vi "CRYGet CurrentSteps By StepNo.vi"(11 "Step Setup VI No":i32) -> (0 "bResult":bool, 2 "Index":i32, 3 "Step":T1={"No.VI"=0, "Category"="", "StepName"="", "Seq setup flattened"="", "Comment"="", "Steps config."=[], "Jump config"=[], "Start"=0.0, "Increment"=0.0, "Name"="Pa", "Unit"="Pa", "Y data"=1, "Y prefix"="", "Y dB ref"=1.0, "Y unit"="", "Repeat State Array"=[]} {"Repeat State Array"."Start" format="%#_5g"; "Y dB ref" format="%.1f"; "Y data" items=["dB", "Lin"]; "Start" format="%#_5g"})   [LabVIEW 2013]
uses:
  CRYSystem/Typedef Control/CRYStep.ctl
  CRYProject Editor Global.vi
  CRYCurveLibrary/Global/CRYCurve Library Global.vi
  CRYSystem/Calibration/SubVI/CRYCal Global.vi
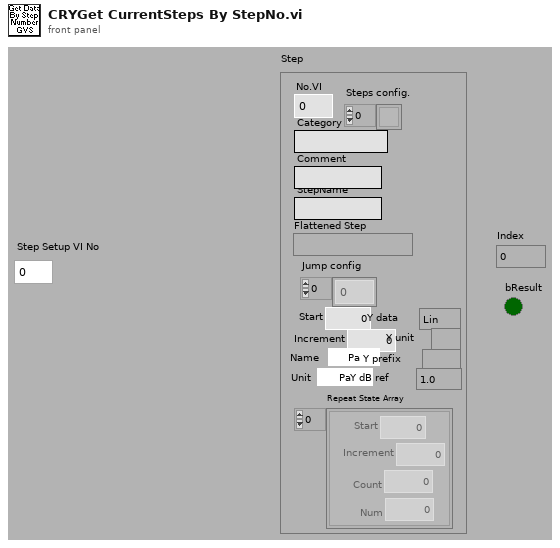
[diagram p1: front panel]
types:
  T1 = typedef "CRYStep.ctl" = cluster{"No.VI":i32, "Category":string, "StepName":string, "Seq setup flattened":string, "Comment":string, "Steps config.":bool[], "Jump config":i32[], "Start":dbl, "Increment":dbl, "Name":string, "Unit":string, "Y data":u16, "Y prefix":string, "Y dB ref":dbl, "Y unit":string, "Repeat State Array":cluster{"Start":dbl, "Increment":dbl, "Count":i32, "Num":i32}[]}
  T2 = typedef "CRYTS.ctl" = cluster{"No.TS":u16, "TS File Path":path, "TS Name":string, "EditStepName":string, "Steps":T1[], "New State":bool, "Change State":bool, "Flattened CurveLib Data":string, "Document Data":string, "EditStepNo":u16, "Operator Start File":string, "Sequence Type":string, "Sequence Language":string}
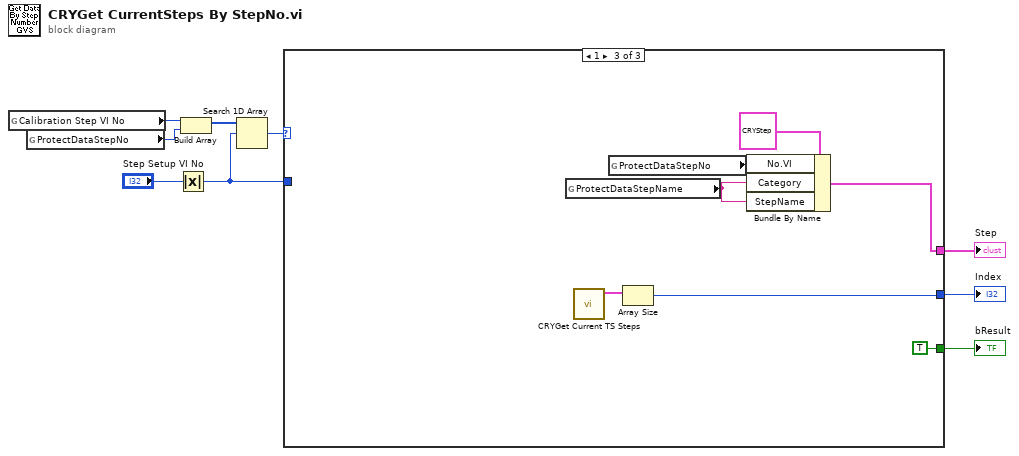
[diagram p0: block diagram]
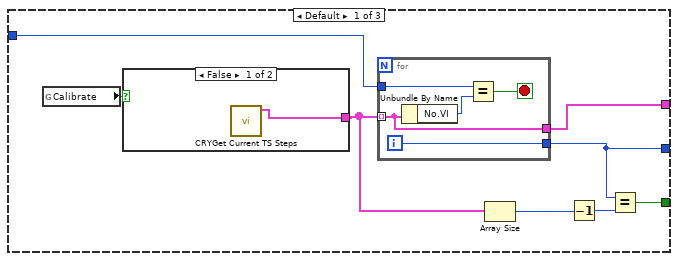
[diagram p2: hidden frame]
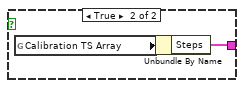
[diagram p3: hidden frame]
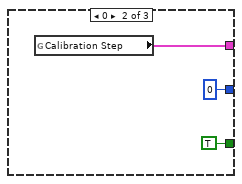
[diagram p4: hidden frame]
diagram:
  n1 = global read "CRYProject Editor Global.vi" "Calibration Step VI No"() -> (w5:i32)
  n2 = global read "CRYCurve Library Global.vi" "ProtectDataStepNo"() -> (w4:i32)
  n3 = Absolute Value(x="Step Setup VI No") -> (abs(x)=w2:i32)
  n4 = Build Array(w5, w4) -> (w3:i32[])
  n5 = Search 1D Array(1D array=w3, element=w2) -> (index of element=w1:i32)  [unwired: 1 in]
  n6 = case shown="1" w1 {
    tunnel: [w16 w28 w30] -> w8
    tunnel: w2 -> [w15 _ _]
    tunnel: [w13 0 w34] -> w7
    tunnel: [w10 TRUE TRUE] -> w6
    frame Default {
      n7 = global read "CRYCal Global.vi" "Calibrate"() -> (w17:bool)
      n8 = case shown="False" w17 {
        tunnel: [w23 w24] -> w14
        frame False {
          n9 = call "CRYGet Current TS Steps.vi"() -> ("Steps"=w23:T1[])  [unwired: 7 in, 4 out]
        }
        frame True {
          n10 = global read "CRYProject Editor Global.vi" "Calibration TS Array"() -> (w25:T2)
          n11 = Unbundle By Name(w25) -> ("Steps"=w24:T1[])
        }
      }
      n12 = for {
        tunnel: w14 -> [w19] mode=indexing
        tunnel: w15 -> [w22]
        tunnel: [w19] -> w16
        tunnel: [w18] -> w13
        i -> [w18]
        stop <- w20 stop-if-true
        n13 = Unbundle By Name(w19) -> ("No.VI"=w21:i32)
        n14 = Equal?(x=w22, y=w21) -> (x = y?=w20:bool)
      }
      n15 = Array Size(array=w14) -> (size(s)=w12:i32)
      n16 = Decrement(x=w12) -> (x-1=w11:i32)
      n17 = Equal?(x=w13, y=w11) -> (x = y?=w10:bool)
    }
    frame 0 {
      n18 = global read "CRYProject Editor Global.vi" "Calibration Step"() -> (w28:T1)
    }
    frame 1 {
      n19 = global read "CRYCurve Library Global.vi" "ProtectDataStepName"() -> (w29:string)
      n20 = call "CRYGet Current TS Steps.vi"() -> ("Steps"=w35:T1[])  [unwired: 7 in, 4 out]
      n21 = global read "CRYCurve Library Global.vi" "ProtectDataStepNo"() -> (w31:i32)
      n22 = Array Size(array=w35) -> (size(s)=w34:i32)
      n23 = Bundle By Name(cluster=T1 {"No.VI"=0, "Category"="", "StepName"="", "Seq setup flattened"="", "Comment"="", "Steps config."=[], "Jump config"=[], "Start"=0.0, "Increment"=0.0, "Name"="Pa", "Unit"="Pa", "Y data"=1, "Y prefix"="", "Y dB ref"=1.0, "Y unit"="", "Repeat State Array"=[]} ("Calibration Step"), "No.VI"=w31, "Category"=w29, "StepName"=w29) -> (w30:T1)
    }
  }
  "Step" <- w8
  "Index" <- w7
  "bResult" <- w6
